vi "Waveform and XY Plots.vi"() -> ()   [LabVIEW 2023]
doc: "Uses the Plot Waveform VI and Plot XY VI to draw a waveform and XY graph in a picture indicator."
panel:
  out "XY Plot":picture
  out "Waveform Plot":picture
  # "Overview: Uses the Plot Waveform VI and the Plot XY VI to draw a waveform and XY graph in a picture indicator.\nInstructions:\nRun the VI."
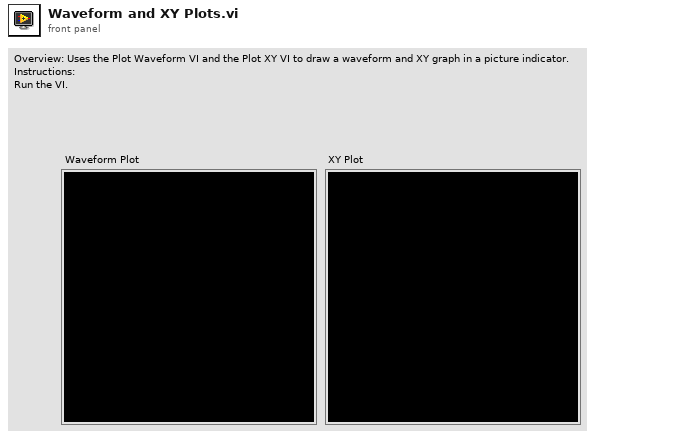
[diagram p1: front panel]
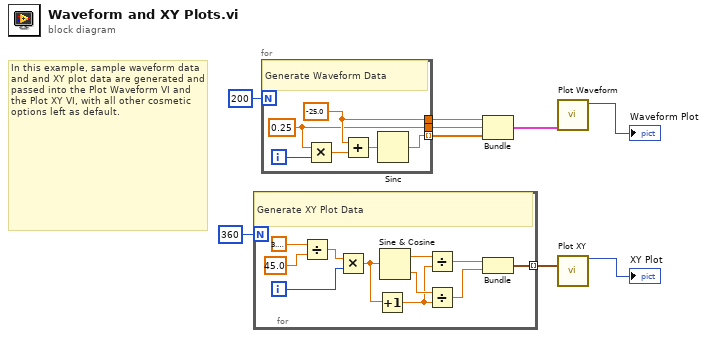
[diagram p0: block diagram]
diagram:
  # "In this example, sample waveform data and and XY plot data are generated and passed into the Plot Waveform VI and the Plot XY VI, with all other cosmetic options left as default."
  n1 = for {
    N: 360 -> [_]
    tunnel: [w20] -> w4 mode=indexing
    i -> [w12]
    # "Generate XY Plot Data"
    n2 = Divide(x=3.141592653589793, y=45.0) -> (x/y=w11:dbl)
    n3 = Multiply(x=w11, y=w12) -> (x*y=w14:dbl)
    n4 = Increment(x=w14) -> (x+1=w13:dbl)
    n5 = Sine & Cosine(0:w14) -> (1:w18:dbl, 2:w16:dbl)
    n6 = Divide(x=w18, y=w13) -> (x/y=w17:dbl)
    n7 = Divide(x=w16, y=w13) -> (x/y=w15:dbl)
    n8 = Bundle(w17, w15) -> (w20:cluster{dbl, dbl})  [unwired: 1 in]
  }
  n9 = for {
    N: 200 -> [_]
    tunnel: [w24] -> w8 mode=indexing
    tunnel: [w22] -> w7
    tunnel: [w21] -> w6
    i -> [w26]
    w21 = 0.25
    w22 = -25.0
    # "Generate Waveform Data"
    n10 = Multiply(x=w21, y=w26) -> (x*y=w25:dbl)
    n11 = Add(x=w22, y=w25) -> (x+y=w23:dbl)
    n12 = Sinc(1:w23) -> (0:w24:dbl)
  }
  n13 = Bundle(w7, w6, w8) -> (w5:cluster{dbl, dbl, dbl[]})  [unwired: 1 in]
  n14 = call <vilib>:"Plot Waveform.vi"("waveform data"=w5) -> ("new picture"=→"Waveform Plot":picture)  [unwired: 10 in]
  n15 = call <vilib>:"Plot XY.vi"("data"=w4) -> ("new picture"=→"XY Plot":picture)  [unwired: 14 in]
